vi "InsertDevDataN.vi"(8 "错误输入":errorcluster, 9 "DevNASSData":T1, 10 "选定检测区域":string, 11 "date/time string":string) -> (0 "错误输出":errorcluster, 1 "数据采集模块地址":string, 2 "detec_electrode_name":string, 3 "elecNum":i32)   [LabVIEW 2014, in "DataBase.lvlib"]
uses:
  DataBase.lvlib
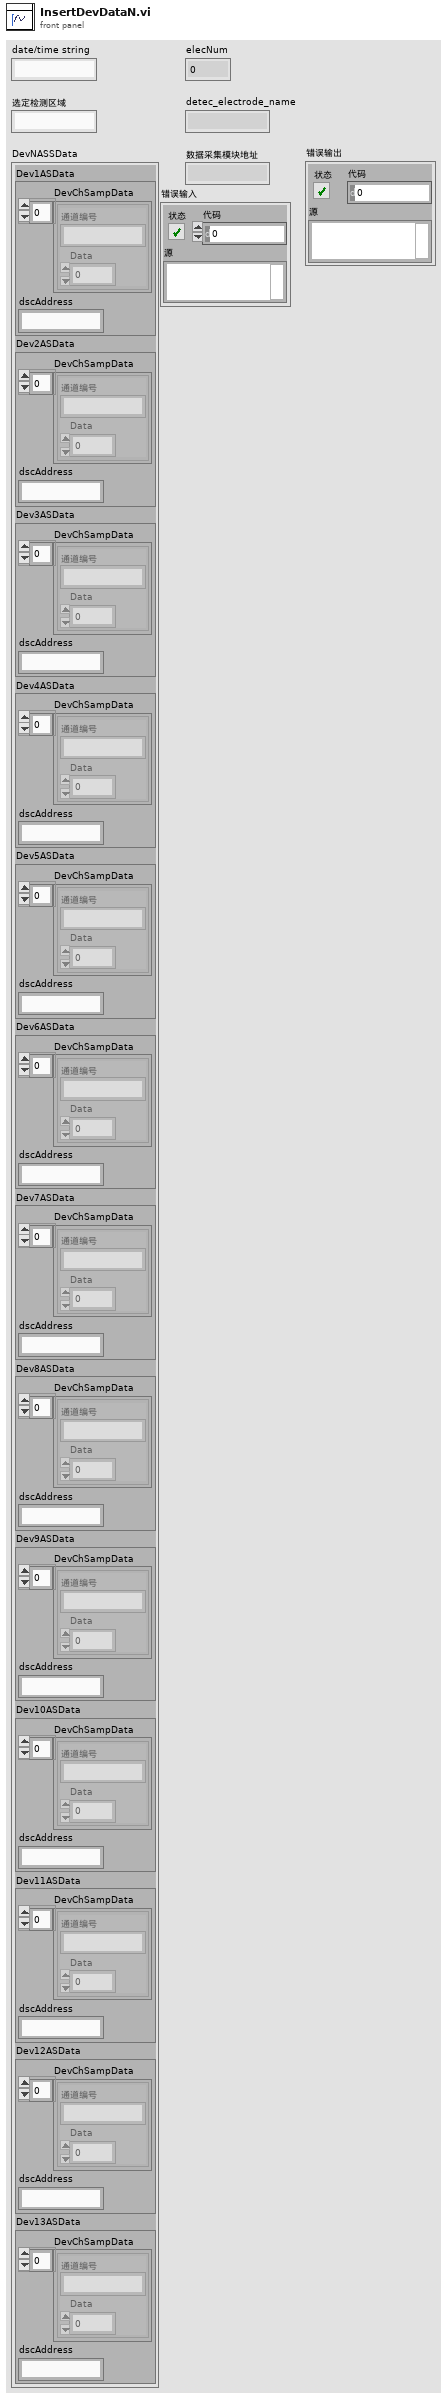
[diagram p1: front panel]
types:
  T1 = cluster{"Dev1ASData":cluster{"DevChSampData":cluster{"通道编号":string, "Data":dbl}[], "dscAddress":string}, "Dev2ASData":cluster{"DevChSampData":cluster{"通道编号":string, "Data":dbl}[], "dscAddress":string}, "Dev3ASData":cluster{"DevChSampData":cluster{"通道编号":string, "Data":dbl}[], "dscAddress":string}, "Dev4ASData":cluster{"DevChSampData":cluster{"通道编号":string, "Data":dbl}[], "dscAddress":string}, "Dev5ASData":cluster{"DevChSampData":cluster{"通道编号":string, "Data":dbl}[], "dscAddress":string}, "Dev6ASData":cluster{"DevChSampData":cluster{"通道编号":string, "Data":dbl}[], "dscAddress":string}, "Dev7ASData":cluster{"DevChSampData":cluster{"通道编号":string, "Data":dbl}[], "dscAddress":string}, "Dev8ASData":cluster{"DevChSampData":cluster{"通道编号":string, "Data":dbl}[], "dscAddress":string}, "Dev9ASData":cluster{"DevChSampData":cluster{"通道编号":string, "Data":dbl}[], "dscAddress":string}, "Dev10ASData":cluster{"DevChSampData":cluster{"通道编号":string, "Data":dbl}[], "dscAddress":string}, "Dev11ASData":cluster{"DevChSampData":cluster{"通道编号":string, "Data":dbl}[], "dscAddress":string}, "Dev12ASData":cluster{"DevChSampData":cluster{"通道编号":string, "Data":dbl}[], "dscAddress":string}, "Dev13ASData":cluster{"DevChSampData":cluster{"通道编号":string, "Data":dbl}[], "dscAddress":string}}
  T2 = cluster{"DevChSampData":cluster{"通道编号":string, "Data":dbl}[], "dscAddress":string}
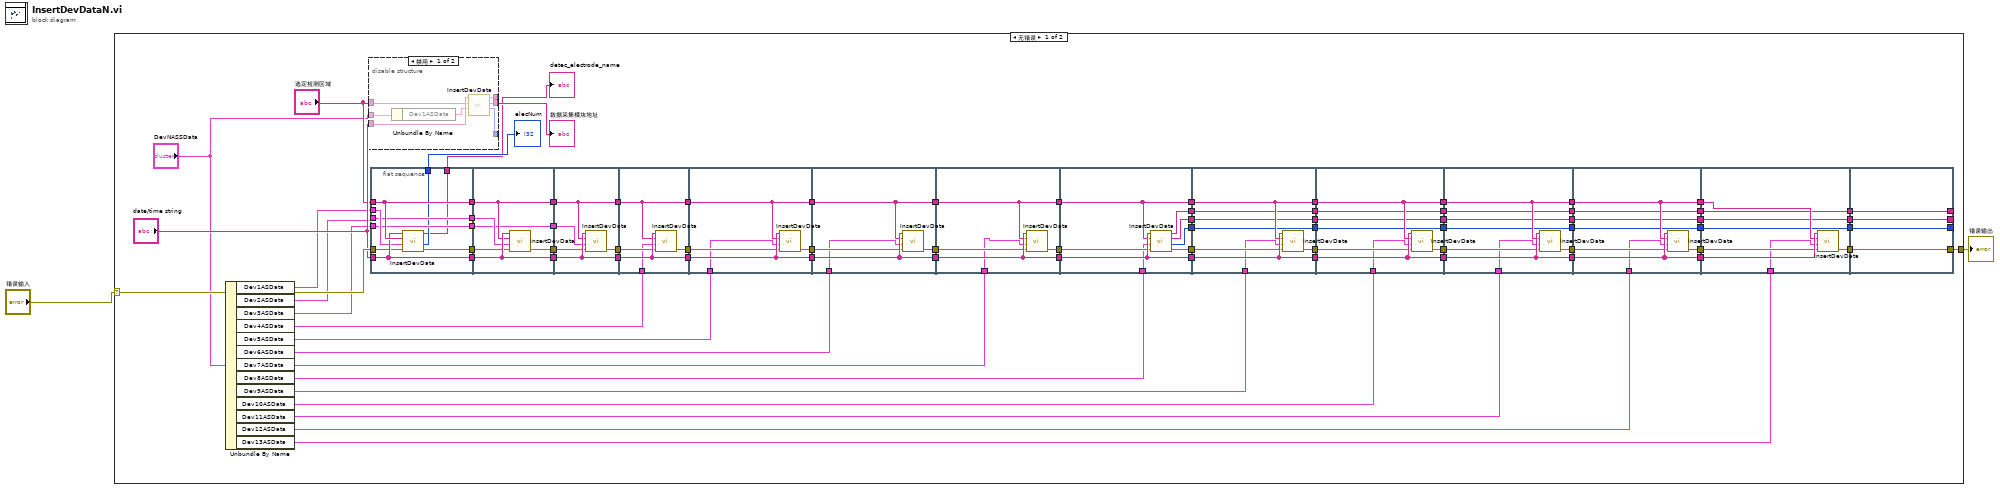
[diagram p0: block diagram]
diagram:
  n1 = case shown="无错误" "错误输入" {
    selector: "错误输入" -> [w81 w181]
    tunnel: [w80 w181] -> w1
    frame No Error {
      n2 = Unbundle By Name("DevNASSData") -> ("Dev1ASData"=w25:T2, "Dev2ASData"=w23:T2, "Dev3ASData"=w22:T2, "Dev4ASData"=w19:T2, "Dev5ASData"=w18:T2, "Dev6ASData"=w17:T2, "Dev7ASData"=w16:T2, "Dev8ASData"=w15:T2, "Dev9ASData"=w14:T2, "Dev10ASData"=w13:T2, "Dev11ASData"=w12:T2, "Dev12ASData"=w11:T2, "Dev13ASData"=w10:T2)
      n3 = disable-structure shown="禁用" {
        disable-tunnel: "date/time string" -> [w88 _]
        disable-tunnel: "选定检测区域" -> [w87 _]
        disable-tunnel: "DevNASSData" -> [w86 _]
        disable-tunnel: [w84 _] -> _
        disable-tunnel: [w83 _] -> w5
        disable-tunnel: [w82 _] -> _
        frame Disabled {
          n4 = Unbundle By Name(w86) -> ("Dev1ASData"=w85:T2)
          n5 = call "InsertDevData.vi"("DevnASData"=w85, "选定检测区域"=w87, "date/time string"=w88) -> ("elecNum"=w82:i32, "数据采集模块地址"=w83:string, "detec_electrode_name"=w84:string)  [unwired: 5 in, 1 out]
        }
        frame Enabled {
        }
      }
      "数据采集模块地址" <- w5
      n6 = flat-sequence {
        tunnel: "选定检测区域" -> [w97]
        tunnel: "date/time string" -> [w96]
        tunnel: w81 -> [w95]
        tunnel: [w97] -> w77
        tunnel: [w96] -> w76
        tunnel: [w94] -> w75
        tunnel: w25 -> [w93]
        tunnel: [w92] -> w24
        tunnel: w23 -> [w92]
        tunnel: w22 -> [w91]
        tunnel: [w91] -> w21
        tunnel: [w90] -> w4
        tunnel: [w89] -> w3
        tunnel: w77 -> [w102]
        tunnel: w76 -> [w103]
        tunnel: w75 -> [w101]
        tunnel: [w102] -> w74
        tunnel: [w103] -> w73
        tunnel: [w100] -> w72
        tunnel: w24 -> [w99]
        tunnel: w21 -> [w98]
        tunnel: [w98] -> w20
        tunnel: w74 -> [w107]
        tunnel: w73 -> [w108]
        tunnel: w72 -> [w106]
        tunnel: [w107] -> w71
        tunnel: [w108] -> w70
        tunnel: [w105] -> w69
        tunnel: w20 -> [w104]
        tunnel: w71 -> [w112]
        tunnel: w70 -> [w113]
        tunnel: w69 -> [w111]
        tunnel: [w112] -> w68
        tunnel: [w113] -> w67
        tunnel: [w110] -> w66
        tunnel: w19 -> [w109]
        tunnel: w68 -> [w115]
        tunnel: w67 -> [w118]
        tunnel: w66 -> [w117]
        tunnel: [w118] -> w65
        tunnel: [w116] -> w64
        tunnel: [w115] -> w63
        tunnel: w18 -> [w114]
        tunnel: w65 -> [w123]
        tunnel: w64 -> [w122]
        tunnel: w63 -> [w121]
        tunnel: [w121] -> w62
        tunnel: [w123] -> w61
        tunnel: [w120] -> w60
        tunnel: w17 -> [w119]
        tunnel: w62 -> [w127]
        tunnel: w61 -> [w128]
        tunnel: w60 -> [w126]
        tunnel: [w127] -> w59
        tunnel: [w128] -> w58
        tunnel: [w125] -> w57
        tunnel: w16 -> [w124]
        tunnel: w59 -> [w135]
        tunnel: w58 -> [w136]
        tunnel: w57 -> [w131]
        tunnel: [w135] -> w56
        tunnel: [w136] -> w55
        tunnel: [w134] -> w54
        tunnel: [w133] -> w53
        tunnel: [w132] -> w52
        tunnel: [w130] -> w51
        tunnel: w15 -> [w129]
        tunnel: w56 -> [w143]
        tunnel: w55 -> [w144]
        tunnel: w54 -> [w140]
        tunnel: w53 -> [w139]
        tunnel: w52 -> [w138]
        tunnel: w51 -> [w142]
        tunnel: [w143] -> w50
        tunnel: [w144] -> w49
        tunnel: [w140] -> w48
        tunnel: [w139] -> w47
        tunnel: [w138] -> w46
        tunnel: [w141] -> w45
        tunnel: w14 -> [w137]
        tunnel: w50 -> [w151]
        tunnel: w49 -> [w152]
        tunnel: w48 -> [w148]
        tunnel: w47 -> [w147]
        tunnel: w46 -> [w146]
        tunnel: w45 -> [w150]
        tunnel: [w151] -> w44
        tunnel: [w152] -> w43
        tunnel: [w148] -> w42
        tunnel: [w147] -> w41
        tunnel: [w146] -> w40
        tunnel: [w149] -> w39
        tunnel: w13 -> [w145]
        tunnel: w44 -> [w159]
        tunnel: w43 -> [w160]
        tunnel: w42 -> [w156]
        tunnel: w41 -> [w155]
        tunnel: w40 -> [w154]
        tunnel: w39 -> [w158]
        tunnel: [w159] -> w38
        tunnel: [w160] -> w37
        tunnel: [w156] -> w36
        tunnel: [w155] -> w35
        tunnel: [w154] -> w34
        tunnel: [w157] -> w33
        tunnel: w12 -> [w153]
        tunnel: w38 -> [w167]
        tunnel: w37 -> [w168]
        tunnel: w36 -> [w164]
        tunnel: w35 -> [w163]
        tunnel: w34 -> [w162]
        tunnel: w33 -> [w166]
        tunnel: [w167] -> w32
        tunnel: [w168] -> w31
        tunnel: [w164] -> w30
        tunnel: [w163] -> w29
        tunnel: [w162] -> w28
        tunnel: [w165] -> w27
        tunnel: w11 -> [w161]
        tunnel: w32 -> [w175]
        tunnel: w31 -> [w176]
        tunnel: w30 -> [w172]
        tunnel: w29 -> [w171]
        tunnel: w28 -> [w170]
        tunnel: w27 -> [w173]
        tunnel: w10 -> [w169]
        tunnel: [w174] -> w9
        tunnel: [w172] -> w8
        tunnel: [w171] -> w7
        tunnel: [w170] -> w6
        tunnel: [w177] -> _
        tunnel: [w178] -> _
        tunnel: [w179] -> _
        tunnel: [w180] -> w80
        tunnel: w9 -> [w180]
        tunnel: w8 -> [w179]
        tunnel: w7 -> [w178]
        tunnel: w6 -> [w177]
        frame #0 {
          n7 = call "InsertDevData.vi"("错误输入"=w95, "DevnASData"=w93, "选定检测区域"=w97, "date/time string"=w96) -> ("错误输出"=w94:errorcluster, "elecNum"=w90:i32, "detec_electrode_name"=w89:string)  [unwired: 4 in, 1 out]
        }
        frame #1 {
          n8 = call "InsertDevData.vi"("错误输入"=w101, "DevnASData"=w99, "选定检测区域"=w102, "date/time string"=w103) -> ("错误输出"=w100:errorcluster)  [unwired: 4 in, 3 out]
        }
        frame #2 {
          n9 = call "InsertDevData.vi"("错误输入"=w106, "DevnASData"=w104, "选定检测区域"=w107, "date/time string"=w108) -> ("错误输出"=w105:errorcluster)  [unwired: 4 in, 3 out]
        }
        frame #3 {
          n10 = call "InsertDevData.vi"("错误输入"=w111, "DevnASData"=w109, "选定检测区域"=w112, "date/time string"=w113) -> ("错误输出"=w110:errorcluster)  [unwired: 4 in, 3 out]
        }
        frame #4 {
          n11 = call "InsertDevData.vi"("错误输入"=w117, "DevnASData"=w114, "选定检测区域"=w115, "date/time string"=w118) -> ("错误输出"=w116:errorcluster)  [unwired: 4 in, 3 out]
        }
        frame #5 {
          n12 = call "InsertDevData.vi"("错误输入"=w122, "DevnASData"=w119, "选定检测区域"=w121, "date/time string"=w123) -> ("错误输出"=w120:errorcluster)  [unwired: 4 in, 3 out]
        }
        frame #6 {
          n13 = call "InsertDevData.vi"("错误输入"=w126, "DevnASData"=w124, "选定检测区域"=w127, "date/time string"=w128) -> ("错误输出"=w125:errorcluster)  [unwired: 4 in, 3 out]
        }
        frame #7 {
          n14 = call "InsertDevData.vi"("错误输入"=w131, "DevnASData"=w129, "选定检测区域"=w135, "date/time string"=w136) -> ("错误输出"=w130:errorcluster, "elecNum"=w132:i32, "数据采集模块地址"=w133:string, "detec_electrode_name"=w134:string)  [unwired: 4 in]
        }
        frame #8 {
          n15 = call "InsertDevData.vi"("错误输入"=w142, "DevnASData"=w137, "选定检测区域"=w143, "date/time string"=w144) -> ("错误输出"=w141:errorcluster)  [unwired: 4 in, 3 out]
        }
        frame #9 {
          n16 = call "InsertDevData.vi"("错误输入"=w150, "DevnASData"=w145, "选定检测区域"=w151, "date/time string"=w152) -> ("错误输出"=w149:errorcluster)  [unwired: 4 in, 3 out]
        }
        frame #10 {
          n17 = call "InsertDevData.vi"("错误输入"=w158, "DevnASData"=w153, "选定检测区域"=w159, "date/time string"=w160) -> ("错误输出"=w157:errorcluster)  [unwired: 4 in, 3 out]
        }
        frame #11 {
          n18 = call "InsertDevData.vi"("错误输入"=w166, "DevnASData"=w161, "选定检测区域"=w167, "date/time string"=w168) -> ("错误输出"=w165:errorcluster)  [unwired: 4 in, 3 out]
        }
        frame #12 {
          n19 = call "InsertDevData.vi"("错误输入"=w173, "DevnASData"=w169, "选定检测区域"=w175, "date/time string"=w176) -> ("错误输出"=w174:errorcluster)  [unwired: 4 in, 3 out]
        }
        frame #13 {
        }
      }
      "elecNum" <- w4
      "detec_electrode_name" <- w3
    }
    frame Error {
    }
  }
  "错误输出" <- w1
